vi "SuperScale - 2-17-2012 (SubVI).vi"(0 "Measured Signals":dbl[](array[numeric]), 11 "Error Input":errorcluster, 13 "Scale Reference":refnum<vi>) -> (4 "Scaled Values":dbl[](array[numeric]), 15 "Scale Error":errorcluster)   [LabVIEW 2011]
uses:
  nilvaiu.dll
  C:/Program Files (x86)/National Instruments/LabVIEW 2011/resource/objmgr/daqmx.rc
panel:
  in  "Scale Template":T1={"Channel Select"=0, "Clear/Reset Scales"=FALSE, "Channel #"=["0", "1", "2"], "Scale Names"=["a", "b", "c"], "Set?"=[FALSE, FALSE, FALSE, FALSE, FALSE, FALSE], "HI/LO Setpoints"=[1.0, 0.0, 1.0, 0.0, 1.0, 0.0], "Units"=["vdc", "vdc", "vdc"], "HI/LO Signals"=[1.0, 0.0, 1.0, 0.0, 1.0, 0.0], "Slope/Intercept"=[1.0, 0.0, 1.0, 0.0, 1.0, 0.0], "IN/OUT Values"=[1.0, 1.0, 2.0, 2.0, 3.0, 3.0], "Sim Signals?"=FALSE, "Sim. Signal"=0.0} {"Sim. Signal" format="%#.3p"; "Channel Select" min=0 step=1; "Slope/Intercept" format="%#.3p"; "HI/LO Setpoints" format="%#.3p"; "IN/OUT Values" format="%#.3p"; "HI/LO Signals" format="%#.3p"}
  # "Super Scale SubVI\nCreated by Blake Otting - Ecolab - 2011"
  # "Instructions:\n1) Create the scale interface below by right-clicking on the Scale Template Input of this SubVI (from your main program) and creating a control.\n2) Create a Reference by right-clicking the on scale interface cluster created in step one.\n3) Connect this Reference to the input of this SubVI along with the Measured (Raw) Signals Array."
  # "Scale Template"
  # "OUTPUTS"
  # "INPUTS"
  # "Ch.\n#"
  # "Scale\nName"
  # "Set\nValues?"
  # "Channel\nSelect"
  # "Scaled"
  # "Pre-Scaled"
  # "Scaling Result"
  # "Values"
  # "Units"
  # "Values"
  # "HI"
  # "Slope"
  # "IN"
  # "LO"
  # "Intercept"
  # "OUT"
  # "HI"
  # "Slope"
  # "IN"
  # "LO"
  # "Intercept"
  # "OUT"
  # "HI"
  # "Slope"
  # "IN"
  # "LO"
  # "Intercept"
  # "OUT"
  # "HI"
  # "Slope"
  # "IN"
  # "LO"
  # "Intercept"
  # "OUT"
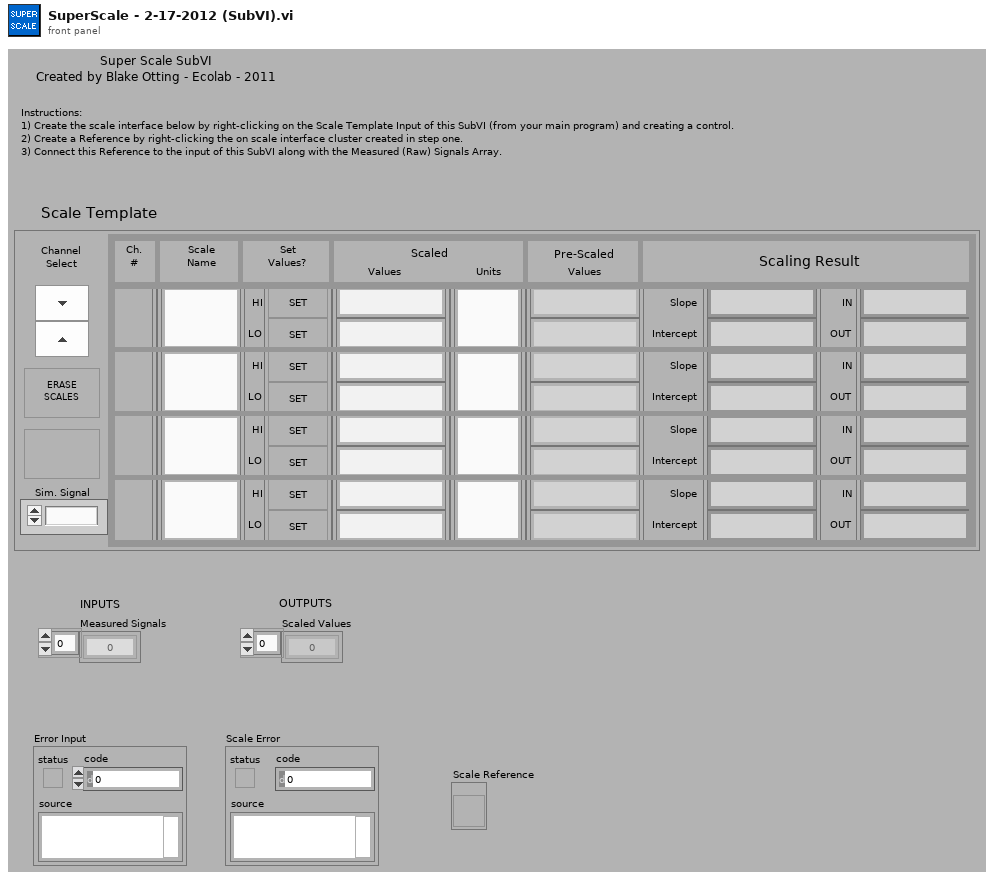
[diagram p1: front panel]
types:
  T1 = cluster{"Channel Select":i32, "Clear/Reset Scales":bool, "Channel #":string[], "Scale Names":string[], "Set?":bool[], "HI/LO Setpoints":dbl[], "Units":string[], "HI/LO Signals":dbl[], "Slope/Intercept":dbl[], "IN/OUT Values":dbl[], "Sim Signals?":bool, "Sim. Signal":dbl}
  T2 = enum16{"open", "replace", "create", "open or create", "replace or create", "replace or create with confirmation"}
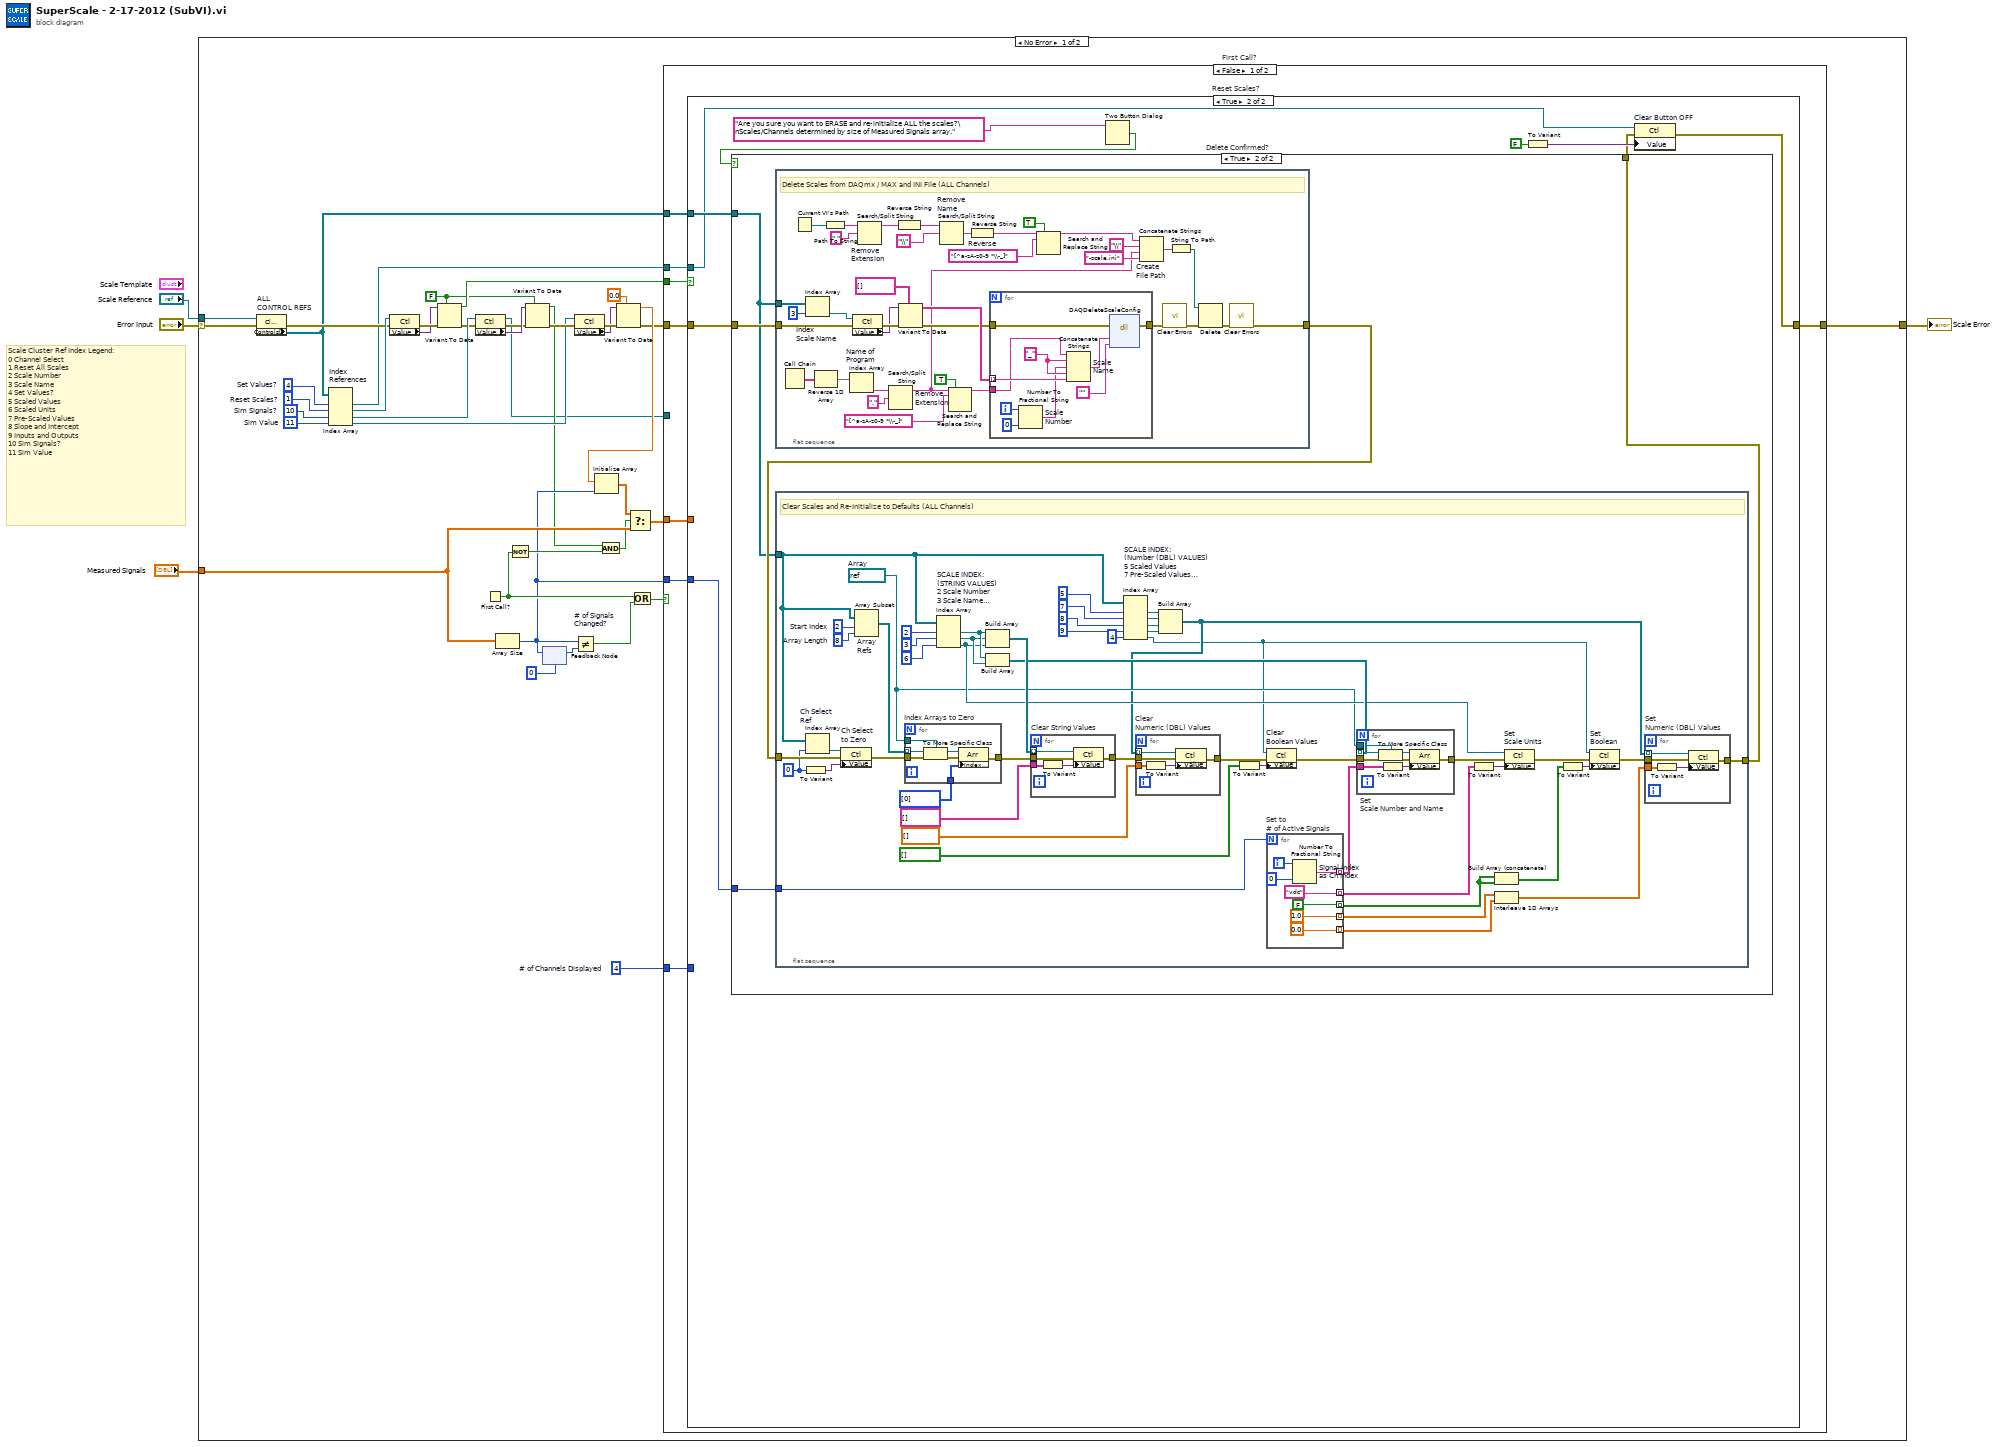
[diagram p0: block diagram]
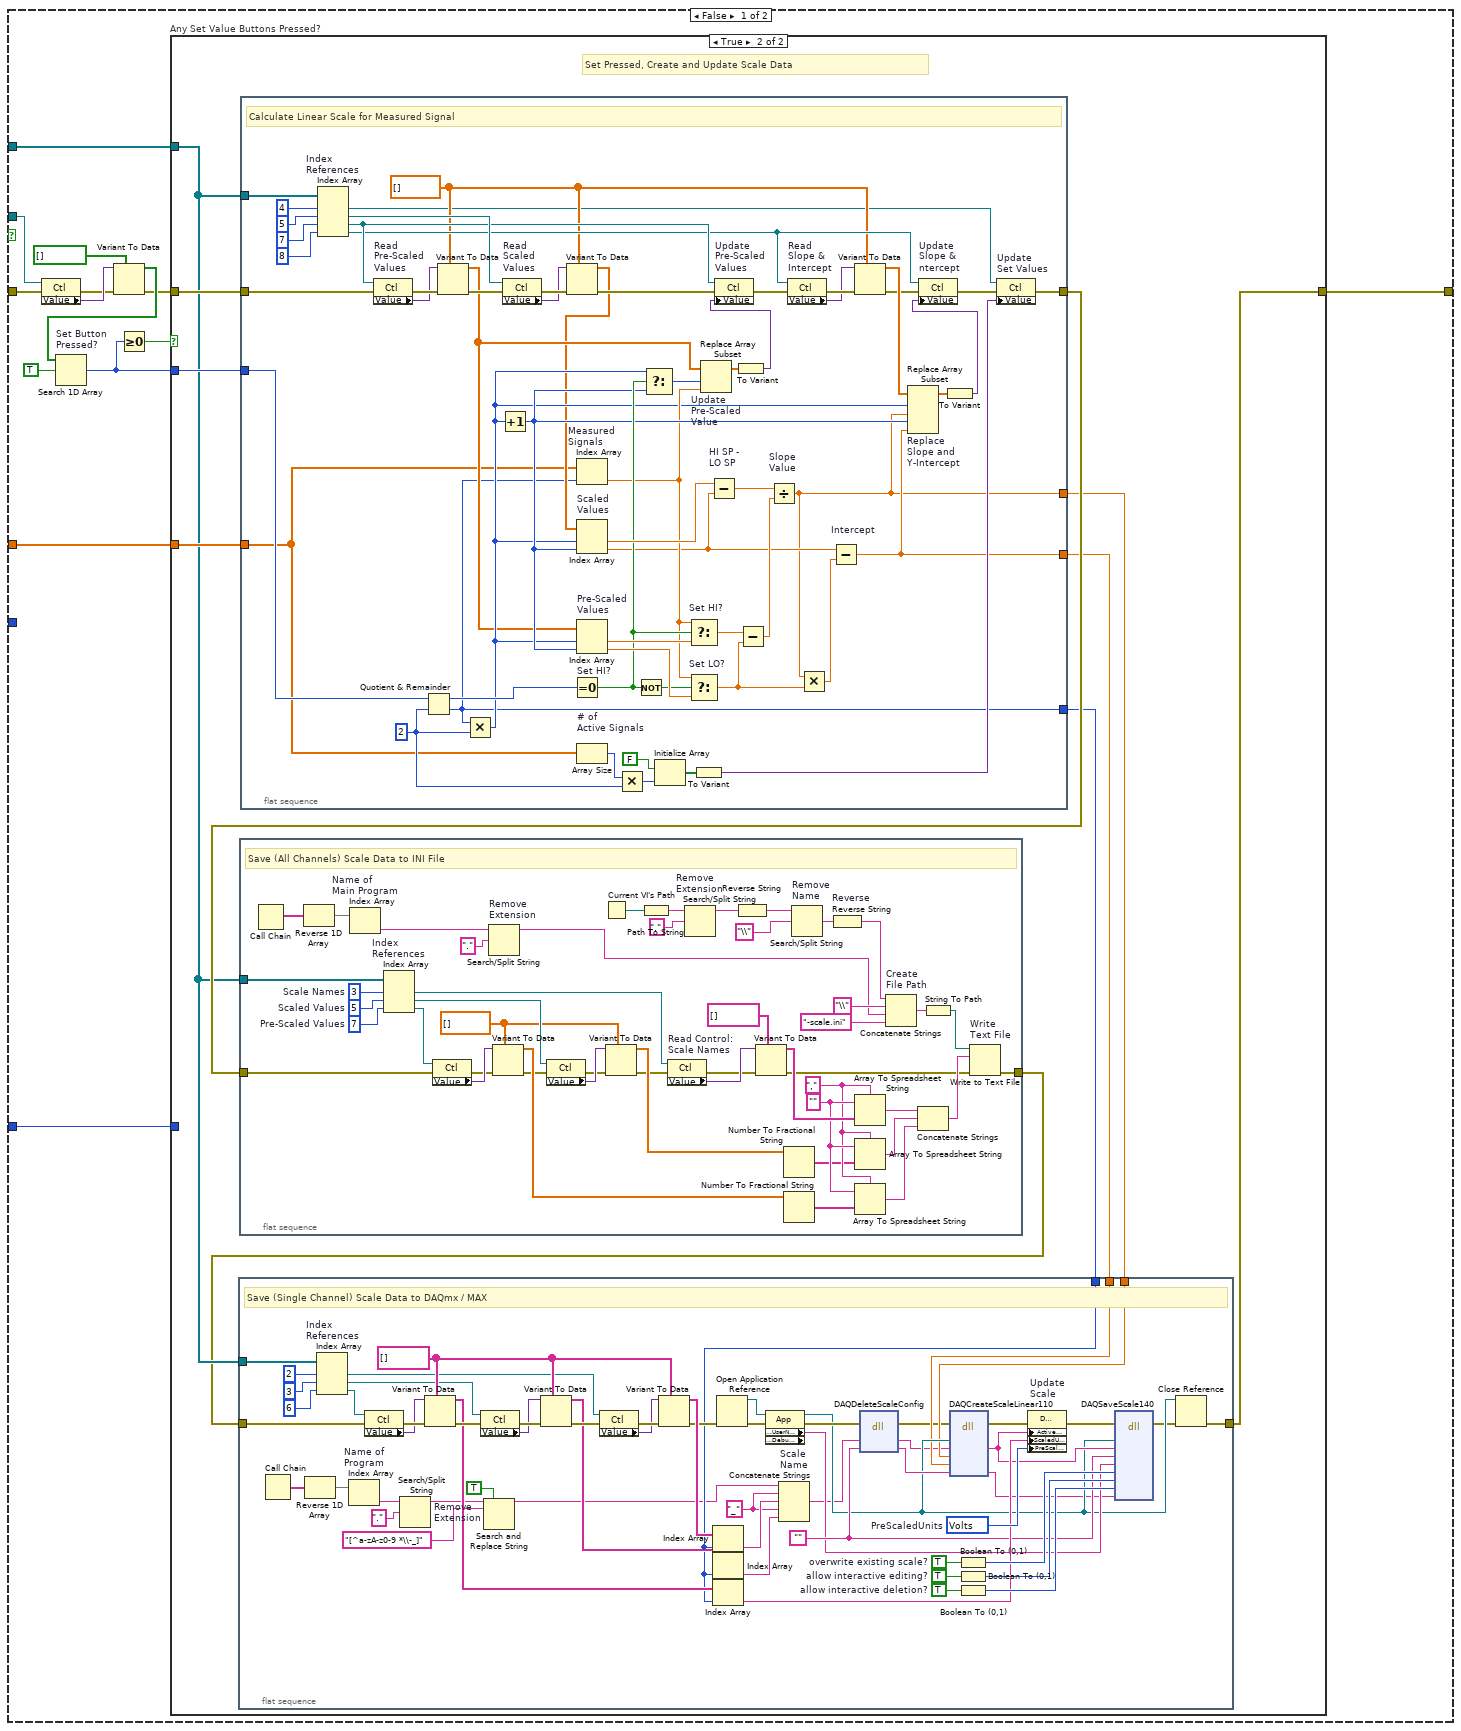
[diagram p2: hidden frame]
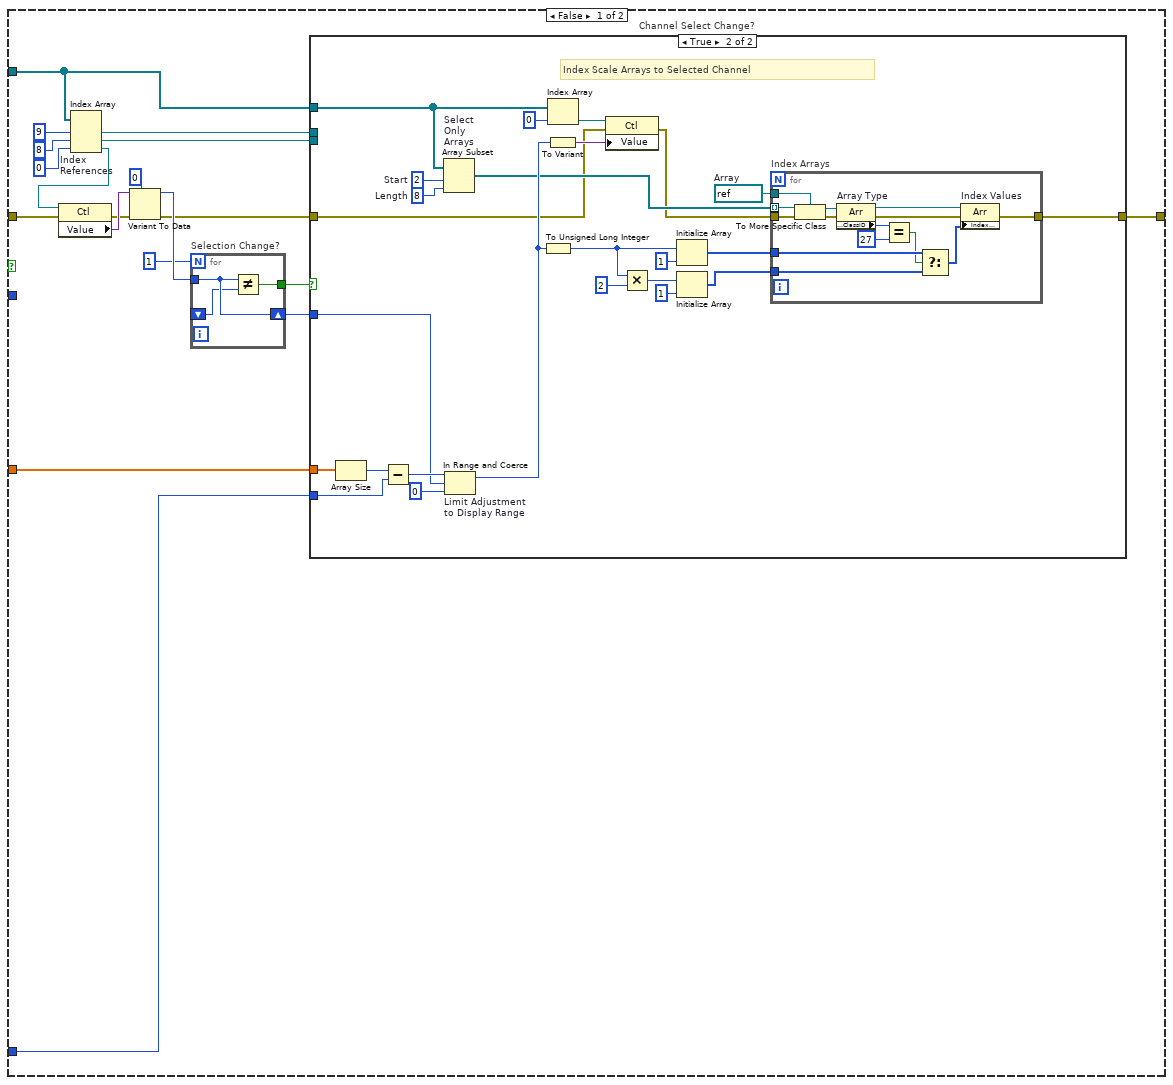
[diagram p3: hidden frame]
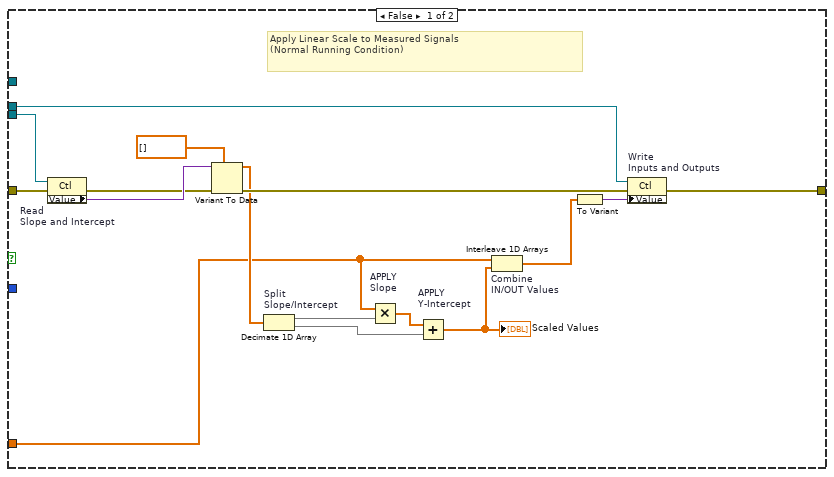
[diagram p4: hidden frame]
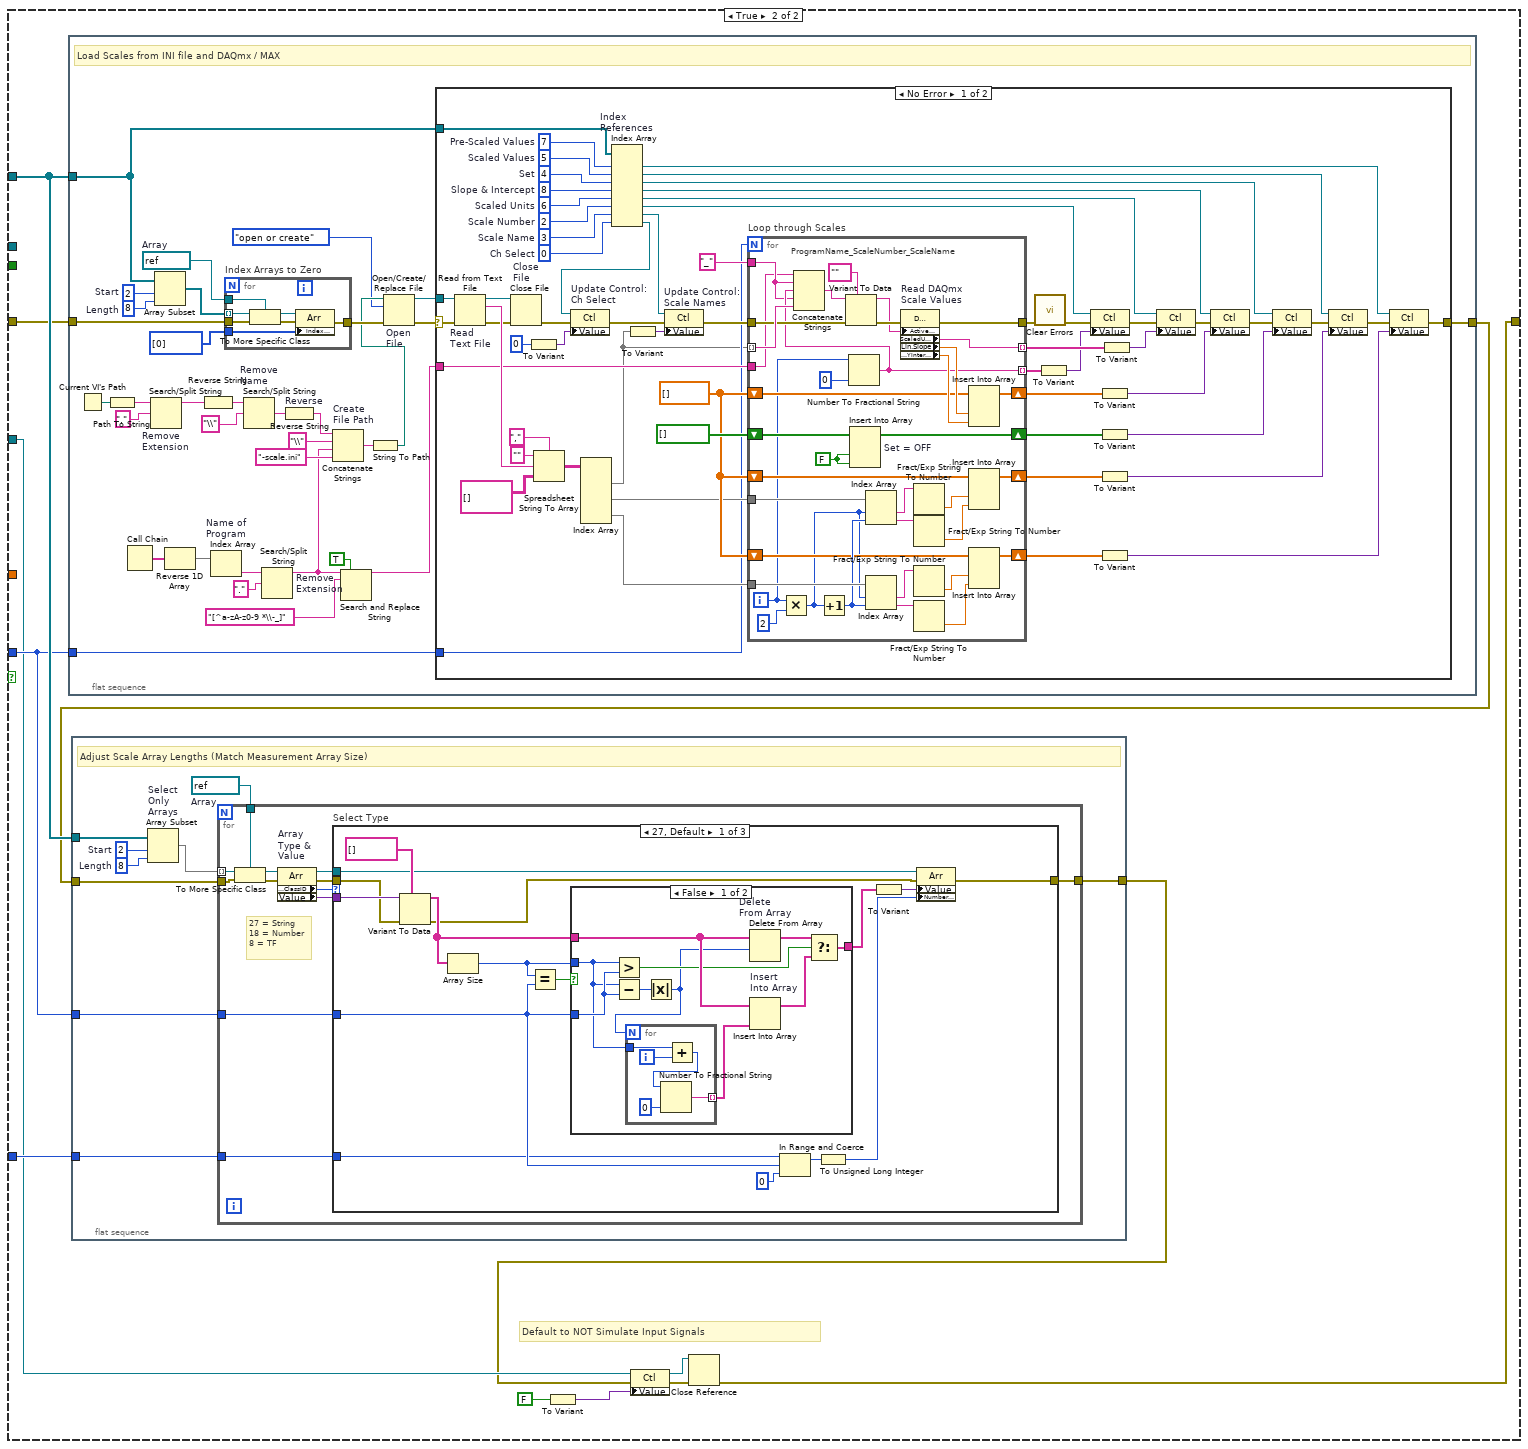
[diagram p6: hidden frame]
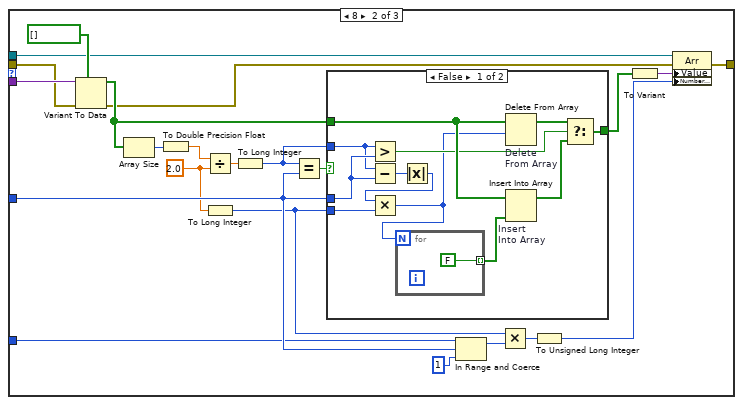
[diagram p8: hidden frame]
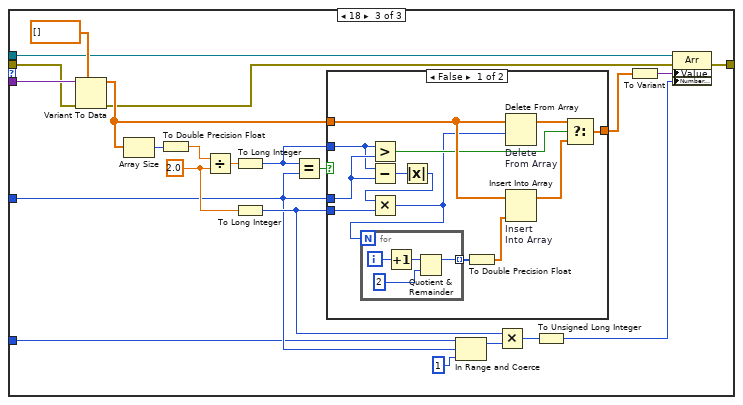
[diagram p10: hidden frame]
diagram:
  # "Scale Cluster Ref Index Legend:\n0 Channel Select\n1 Reset All Scales\n2 Scale Number\n3 Scale Name\n4 Set Values?\n5 Scaled Values\n6 Scaled Units\n7 Pre-Scaled Values\n8 Slope and Intercept\n9 Inputs and Outputs\n10 Sim Signals?\n11 Sim Value"
  n1 = case shown="No Error" "Error Input" {
    selector: "Error Input" -> [w28 w748]
    tunnel: "Scale Reference" -> [w38 _]
    tunnel: "Measured Signals" -> [w25 _]
    tunnel: [w29 w748] -> w3
    frame No Error {
      w19 = 11  # Sim Value
      w20 = 10  # Sim Signals?
      w30 = 4  # Set Values?
      w36 = 4  # # of Channels Displayed
      w14 = FALSE
      w44 = 1  # Reset Scales?
      n2 = property on="ALL\nCONTROL REFS" class="Clust (strict)"(reference=w38, error in=w28) -> (error out=w40:errorcluster, "Controls[]"=w37:refnum<vi>[])  [unwired: 1 out]
      n3 = Index Array "Index\nReferences"(array=w37, index #1=w30, index #2=w44, index #3=w20, index #4=w19) -> (element #1=w31:refnum<vi>, element #2=w43:refnum<vi>, element #3=w18:refnum<vi>, element #4=w8:refnum<vi>)
      n4 = property class="Ctl"(reference=w43, error in=w40) -> (error out=w42:errorcluster, "Value"=w41:variant)  [unwired: 1 out]
      n5 = Variant To Data(error in=w42, type=w14, Variant=w41) -> (data=w39:bool, error out=w17:errorcluster)
      n6 = property class="Ctl"(reference=w18, error in=w17) -> (reference out=w5:refnum<vi>, error out=w15:errorcluster, "Value"=w16:variant)
      n7 = First Call?() -> (First Call?: T/F=w26:bool)
      n8 = Array Size(array=w25) -> (size(s)=w23:i32)
      n9 = Not(x=w26) -> (.not. x?=w27:bool)
      n10 = Variant To Data(error in=w15, type=w14, Variant=w16) -> (data=w6:bool, error out=w9:errorcluster)
      n11 = feedback #1(0) -> (w34:i32)
      n12 = feedback-in #1(w23) -> ()
      n13 = Not Equal? "# of Signals\nChanged?"(x=w23, y=w34) -> (x != y?=w33:bool)
      n14 = property class="Ctl"(reference=w8, error in=w9) -> (error out=w13:errorcluster, "Value"=w7:variant)  [unwired: 1 out]
      n15 = And(x=w6, y=w27) -> (x .and. y?=w21:bool)
      n16 = Variant To Data(error in=w13, type=0.0 ("Simulated Signal"), Variant=w7) -> (data=w11:dbl, error out=w10:errorcluster)
      n17 = Initialize Array(w11, w23) -> (w22:dbl[])
      n18 = Select(t=w22, s=w21, f=w25) -> (s? t:f=w24:dbl[])
      n19 = Or(x=w26, y=w33) -> (x .or. y?=w32:bool)
      n20 = case "First Call?" shown="False" w32 {
        tunnel: w24 -> [w52 _]
        tunnel: w39 -> [w51 _]
        tunnel: w37 -> [w47 w480]
        tunnel: w10 -> [w50 w479]
        tunnel: [w49 w470] -> w29
        tunnel: w36 -> [w48 w478]
        tunnel: w23 -> [w46 w476]
        tunnel: w31 -> [w45 _]
        tunnel: w5 -> [_ w475]
        frame False {
          n21 = case "Reset Scales?" shown="True" w51 {
            tunnel: w47 -> [w55 w321]
            tunnel: w52 -> [w60 _]
            tunnel: w50 -> [w57 w320]
            tunnel: [w56 w325] -> w49
            tunnel: w48 -> [w54 _]
            tunnel: w46 -> [_ w319]
            tunnel: w45 -> [w53 w318]
            frame False {
              n22 = property class="Ctl"(reference=w53, error in=w57) -> (error out=w59:errorcluster, "Value"=w65:variant)  [unwired: 1 out]
              n23 = Variant To Data(error in=w59, type=bool[] [], Variant=w65) -> (data=w63:bool[], error out=w58:errorcluster)
              n24 = Search 1D Array "Set Button\nPressed?"(1D array=w63, element=TRUE) -> (index of element=w61:i32)  [unwired: 1 in]
              n25 = Greater Or Equal To 0?(x=w61) -> (x >= 0?=w62:bool)
              n26 = case "Any Set Value Buttons Pressed?" shown="True" w62 {
                tunnel: w55 -> [w73 w145]
                tunnel: w61 -> [_ w153]
                tunnel: w60 -> [w78 w152]
                tunnel: w58 -> [w77 w151]
                tunnel: [w76 w149] -> w56
                tunnel: w54 -> [w72 _]
                frame False {
                  n27 = Index Array "Index\nReferences"(array=w73, index #1=9, index #2=8, index #3=0) -> (element #1=w68:refnum<vi>, element #2=w71:refnum<vi>, element #3=w74:refnum<vi>)
                  n28 = property class="Ctl"(reference=w74, error in=w77) -> (error out=w83:errorcluster, "Value"=w85:variant)  [unwired: 1 out]
                  n29 = Variant To Data(error in=w83, type=0, Variant=w85) -> (data=w82:i32, error out=w67:errorcluster)
                  n30 = for "Selection Change?" {
                    N: 1 -> [_]
                    tunnel: w82 -> [w143]
                    shift-right: [w143] -> w80
                    shift-left: _ -> [w142]
                    tunnel: [w141] -> w79
                    n31 = Not Equal?(x=w143, y=w142) -> (x != y?=w141:bool)
                  }
                  n32 = case "Channel Select Change?" shown="True" w79 {
                    tunnel: w80 -> [_ w123]
                    tunnel: w67 -> [w101 w103]
                    tunnel: w73 -> [_ w109]
                    tunnel: w78 -> [w88 w122]
                    tunnel: [w100 w104] -> w76
                    tunnel: w72 -> [_ w120]
                    tunnel: w71 -> [w87 _]
                    tunnel: w68 -> [w86 _]
                    frame False {
                      # "Apply Linear Scale to Measured Signals\n(Normal Running Condition)"
                      n33 = property on="Read\nSlope and Intercept" class="Ctl"(reference=w87, error in=w101) -> (error out=w98:errorcluster, "Value"=w99:variant)  [unwired: 1 out]
                      n34 = Variant To Data(error in=w98, type=dbl[] [], Variant=w99) -> (data=w89:dbl[], error out=w90:errorcluster)
                      n35 = Decimate 1D Array "Split\nSlope/Intercept"(w89) -> (w94:dbl[], w95:dbl[])
                      n36 = Multiply "APPLY\nSlope"(x=w88, y=w94) -> (x*y=w96:dbl[])
                      n37 = Add "APPLY\nY-Intercept"(x=w96, y=w95) -> (x+y=w93:dbl[])
                      "Scaled Values" <- w93
                      n38 = Interleave 1D Arrays "Combine\nIN/OUT Values"(w88, w93) -> (w91:dbl[])
                      n39 = To Variant(anything=w91) -> (Variant=w92:variant)
                      n40 = property on="Write\nInputs and Outputs" class="Ctl"(reference=w86, error in=w90, "Value"=w92) -> (error out=w100:errorcluster)  [unwired: 1 out]
                    }
                    frame True {
                      w111 = 8  # Length
                      w110 = 2  # Start
                      w108 = refnum<vi> refnum  # Array
                      # "Index Scale Arrays to Selected Channel"
                      n41 = Array Size(array=w122) -> (size(s)=w121:i32)
                      n42 = Subtract(x=w121, y=w120) -> (x-y=w124:i32)
                      n43 = Array Subset "Select\nOnly \nArrays"(array=w109, index=w110, length=w111) -> (w107:refnum<vi>[])
                      n44 = In Range and Coerce "Limit Adjustment\nto Display Range"(upper limit=w124, x=w123, lower limit=0) -> (coerced(x)=w117:i32)  [unwired: 1 out]
                      n45 = To Unsigned Long Integer(number=w117) -> (unsigned 32bit integer=w114:u32)
                      n46 = Index Array(array=w109, index=0) -> (element=w118:refnum<vi>)
                      n47 = To Variant(anything=w117) -> (Variant=w116:variant)
                      n48 = property class="Ctl"(reference=w118, error in=w103, "Value"=w116) -> (error out=w102:errorcluster)  [unwired: 1 out]
                      n49 = Multiply(x=w114, y=u32 2) -> (x*y=w112:u32)
                      n50 = Initialize Array(w114, 1 ("dimension size")) -> (w106:u32[])
                      n51 = Initialize Array(w112, 1 ("dimension size")) -> (w105:u32[])
                      n52 = for "Index Arrays" {
                        tunnel: w107 -> [w140] mode=indexing
                        tunnel: [w127] -> w104
                        tunnel: w108 -> [w139]
                        tunnel: w102 -> [w138]
                        tunnel: w106 -> [w137]
                        tunnel: w105 -> [w136]
                        n53 = To More Specific Class(target class=w139, reference=w140, error in=w138) -> (specific class reference=w132:refnum<vi>, error out=w133:errorcluster)
                        n54 = property on="Array Type" class="Arr"(reference=w132, error in=w133) -> (reference out=w131:refnum<vi>, error out=w130:errorcluster, "Array Element.ClassID"=w134:u32)
                        n55 = Equal?(x=w134, y=u32 27) -> (x = y?=w128:bool)
                        n56 = Select(t=w137, s=w128, f=w136) -> (s? t:f=w129:u32[])
                        n57 = property on="Index Values" class="Arr"(reference=w131, error in=w130, "Index Values"=w129) -> (error out=w127:errorcluster)  [unwired: 1 out]
                      }
                    }
                  }
                }
                frame True {
                  # "Set Pressed, Create and Update Scale Data"
                  n58 = flat-sequence {
                    tunnel: w145 -> [w240]
                    tunnel: w147 -> [w223]
                    tunnel: w148 -> [w222]
                    tunnel: [w229] -> w149
                    tunnel: w144 -> [w228]
                    tunnel: w146 -> [w221]
                    frame #0 {
                      w254 = string[] []
                      w268 = TRUE  # allow interactive deletion?
                      w267 = TRUE  # allow interactive editing?
                      w266 = TRUE  # overwrite existing scale?
                      w269 = 10348 items=["Volts"=10348, "Amps"=10342, "Deg F"=10144, "Deg C"=10143, "Deg R"=10145, "Kelvins"=10325, "Strain"=10299, "Ohms"=10384, "Hz"=10373, "Seconds"=10364, "Meters"=10219, "Inches"=10379, "Degrees"=10146, "Radians"=10273, "g"=10186, "m/s^2"=12470, "Pascals"=10081, "Newtons"=15875, "Pounds"=15876, "kgf"=15877, "psi"=15879, "bar"=15880, "Nm"=15881, "oz-in"=15882, "lb-in"=15883, "lb-ft"=15884, "Volts/Volt"=15896, "mVolts/Volt"=15897, "From TEDS"=12516]  # PreScaledUnits
                      w238 = ""
                      w234 = "_"
                      # "Save (Single Channel) Scale Data to DAQmx / MAX"
                      n59 = Call Chain() -> (call chain=w225:string[])
                      n60 = Reverse 1D Array(array=w225) -> (reversed array=w224:string[])
                      n61 = Index Array "Index\nReferences"(array=w240, index #1=2, index #2=3, index #3=6) -> (element #1=w251:refnum<vi>, element #2=w250:refnum<vi>, element #3=w249:refnum<vi>)
                      n62 = Index Array "Name of\nProgram"(array=w224) -> (element=w226:string)  [unwired: 1 in]
                      n63 = property class="Ctl"(reference=w249, error in=w228) -> (error out=w259:errorcluster, "Value"=w232:variant)  [unwired: 1 out]
                      n64 = Search/Split String "Remove \nExtension"(string=w226, search string/char (-)=".") -> (substring before match=w213:string)  [unwired: 1 in, 2 out]
                      n65 = Variant To Data(error in=w259, type=w254, Variant=w232) -> (data=w246:string[], error out=w258:errorcluster)
                      n66 = property class="Ctl"(reference=w250, error in=w258) -> (error out=w257:errorcluster, "Value"=w253:variant)  [unwired: 1 out]
                      n67 = Search and Replace String(replace all?=TRUE ("replace all? (F)"), input string=w213, search string="[^a-zA-z0-9 *\\-_]") -> (result string=w214:string)  [unwired: 5 in, 3 out]
                      n68 = Variant To Data(error in=w257, type=w254, Variant=w253) -> (data=w247:string[], error out=w256:errorcluster)
                      n69 = property class="Ctl"(reference=w251, error in=w256) -> (error out=w255:errorcluster, "Value"=w252:variant)  [unwired: 1 out]
                      n70 = Variant To Data(error in=w255, type=w254, Variant=w252) -> (data=w248:string[], error out=w236:errorcluster)
                      n71 = Index Array(array=w248, index=w221) -> (element=w245:string)
                      n72 = Index Array(array=w247, index=w221) -> (element=w244:string)
                      n73 = Index Array(array=w246, index=w221) -> (element=w243:string)
                      n74 = Open Application Reference(8:w236) -> (0:w235:errorcluster, 3:w242:refnum<vi>)  [unwired: 3 in]
                      n75 = property class="App" props=["App.UserName", "App.DebugName"](reference=w242, error in=w235) -> (reference out=w231:refnum<vi>, error out=w237:errorcluster, "App.UserName"=w233:string)  [unwired: 1 out]
                      n76 = Concatenate Strings "Scale\nName"(w214, w234, w245, w234, w244) -> (w216:string)
                      n77 = dll-call lib="nilvaiu.dll" fn="DAQDeleteScaleConfig" label="Delete\nScale"(error in=w237, "scaleName"=w216, "extendedErrorInfo"=w238) -> (error out=w220:errorcluster, "scaleName"=w217:string, "extendedErrorInfo"=w239:string)  [unwired: 3 in, 1 out]
                      n78 = dll-call lib="nilvaiu.*" fn="DAQCreateScaleLinear110" label="Create\nScale"(error in=w220, "This Application"=w231, "name"=w217, "slope"=w222, "yIntercept"=w223, "exterr"=w239) -> (error out=w211:errorcluster, "name"=w241:string, "exterr"=w218:string)  [unwired: 6 in, 1 out]
                      n79 = Boolean To (0,1)(Boolean=w266) -> (0, 1=w265:i16)
                      n80 = Boolean To (0,1)(Boolean=w267) -> (0, 1=w264:i16)
                      n81 = Boolean To (0,1)(Boolean=w268) -> (0, 1=w263:i16)
                      n82 = property on="Update\nScale" class="DAQmx Scale"(error in=w211, "Active Scale"=w241, "ScaledUnits"=w243, "PreScaledUnits"=w269) -> (error out=w219:errorcluster)  [unwired: 1 in, 1 out]
                      n83 = dll-call lib="nilvaiu.*" fn="DAQSaveScale140" label="Save\nScale"(error in=w219, "This Application"=w231, "scaleName"=w241, "saveAs"=w238, "author"=w233, "overwriteMode"=w265, "allowInteractiveEditing?"=w264, "allowInteractiveDeletion?"=w263, "extendedErrorInfo"=w218) -> (error out=w230:errorcluster)  [unwired: 11 in, 1 out]
                      n84 = Close Reference(reference=w231, error in (no error)=w230) -> (error out=w229:errorcluster)
                    }
                  }
                  n85 = flat-sequence {
                    tunnel: w145 -> [w317]
                    tunnel: w150 -> [w316]
                    tunnel: [w315] -> w144
                    frame #0 {
                      w289 = 5  # Scaled Values
                      w290 = 3  # Scale Names
                      w288 = 7  # Pre-Scaled Values
                      w277 = dbl[] [] ("array 2")
                      w302 = "" ("format string")
                      w300 = ","
                      # "Save (All Channels) Scale Data to INI File"
                      n86 = Call Chain() -> (call chain=w273:string[])
                      n87 = Reverse 1D Array(array=w273) -> (reversed array=w272:string[])
                      n88 = Index Array "Name of\nMain Program"(array=w272) -> (element=w274:string)  [unwired: 1 in]
                      n89 = Index Array "Index\nReferences"(array=w317, index #1=w290, index #2=w289, index #3=w288) -> (element #1=w293:refnum<vi>, element #2=w292:refnum<vi>, element #3=w291:refnum<vi>)
                      n90 = property on="Read Control:\nPre-Scaled" class="Ctl"(reference=w291, error in=w316) -> (error out=w310:errorcluster, "Value"=w311:variant)  [unwired: 1 out]
                      n91 = Search/Split String "Remove \nExtension"(string=w274, search string/char (-)=".") -> (substring before match=w271:string)  [unwired: 1 in, 2 out]
                      n92 = Variant To Data(error in=w310, type=w277, Variant=w311) -> (data=w313:dbl[], error out=w312:errorcluster)
                      n93 = property on="Read Control:\nScaled" class="Ctl"(reference=w292, error in=w312) -> (error out=w307:errorcluster, "Value"=w309:variant)  [unwired: 1 out]
                      n94 = Current VI's Path() -> (path=w286:path)
                      n95 = Variant To Data(error in=w307, type=w277, Variant=w309) -> (data=w314:dbl[], error out=w308:errorcluster)
                      n96 = Path To String(path=w286) -> (string=w281:string)
                      n97 = property on="Read Control:\nScale Names" class="Ctl"(reference=w293, error in=w308) -> (error out=w294:errorcluster, "Value"=w296:variant)  [unwired: 1 out]
                      n98 = Search/Split String "Remove \nExtension"(string=w281, search string/char (-)=".") -> (substring before match=w282:string)  [unwired: 1 in, 2 out]
                      n99 = Reverse String ("Reverse")(1:w282) -> (0:w283:string)
                      n100 = Variant To Data(error in=w294, type=string[] [], Variant=w296) -> (data=w305:string[], error out=w304:errorcluster)
                      n101 = Number To Fractional String(number=w314) -> (F-format string=w299:string[])  [unwired: 3 in]
                      n102 = Number To Fractional String(number=w313) -> (F-format string=w303:string[])  [unwired: 3 in]
                      n103 = Search/Split String "Remove\nName"(string=w283, search string/char (-)="\\") -> (match + rest of string=w285:string)  [unwired: 1 in, 2 out]
                      n104 = Reverse String "Reverse"(1:w285) -> (0:w270:string)
                      n105 = Array To Spreadsheet String(delimiter (Tab)=w300, array=w305, 3:w302) -> (spreadsheet string=w297:string)
                      n106 = Array To Spreadsheet String(delimiter (Tab)=w300, array=w299, 3:w302) -> (spreadsheet string=w298:string)
                      n107 = Array To Spreadsheet String(delimiter (Tab)=w300, array=w303, 3:w302) -> (spreadsheet string=w301:string)
                      n108 = Concatenate Strings "Create\nFile Path"(w270, "\\", w271, "-scale.ini") -> (w279:string)
                      n109 = Concatenate Strings(w297, w298, w301) -> (w306:string)
                      n110 = String To Path(string=w279) -> (path=w278:path)
                      n111 = Write to Text File "Write\nText File"(file (use dialog)=w278, text=w306, error in=w304) -> (error out=w315:errorcluster)  [unwired: 1 in, 2 out]
                    }
                  }
                  n112 = flat-sequence {
                    tunnel: w153 -> [w191]
                    tunnel: w152 -> [w160]
                    tunnel: w151 -> [w159]
                    tunnel: [w173] -> w150
                    tunnel: [w154] -> w148
                    tunnel: [w162] -> w147
                    tunnel: [w161] -> w146
                    tunnel: w145 -> [w157]
                    frame #0 {
                      w163 = dbl[] []
                      w166 = 2
                      # "Calculate Linear Scale for Measured Signal"
                      n113 = Index Array "Index\nReferences"(array=w157, index #1=4, index #2=5, index #3=7, index #4=8) -> (element #1=w158:refnum<vi>, element #2=w183:refnum<vi>, element #3=w182:refnum<vi>, element #4=w176:refnum<vi>)
                      n114 = property on="Read\nPre-Scaled\nValues" class="Ctl"(reference=w182, error in=w159) -> (error out=w187:errorcluster, "Value"=w186:variant)  [unwired: 1 out]
                      n115 = Quotient & Remainder(x=w191, y=w166) -> (x-y*floor(x/y)=w194:i32, floor(x/y)=w161:i32)
                      n116 = Variant To Data(error in=w187, type=w163, Variant=w186) -> (data=w165:dbl[], error out=w170:errorcluster)
                      n117 = Multiply(x=w161, y=w166) -> (x*y=w167:i32)
                      n118 = Increment(x=w167) -> (x+1=w198:i32)
                      n119 = property on="Read\nScaled\nValues" class="Ctl"(reference=w183, error in=w170) -> (error out=w185:errorcluster, "Value"=w184:variant)  [unwired: 1 out]
                      n120 = Variant To Data(error in=w185, type=w163, Variant=w184) -> (data=w164:dbl[], error out=w169:errorcluster)
                      n121 = Equal To 0? "Set HI?"(x=w194) -> (x = 0?=w199:bool)
                      n122 = Index Array "Measured\nSignals"(array=w160, index=w161) -> (element=w196:dbl)
                      n123 = Index Array "Scaled\nValues"(array=w164, index #1=w167, index #2=w198) -> (element #1=w210:dbl, element #2=w155:dbl)
                      n124 = Index Array "Pre-Scaled\nValues"(array=w165, index #1=w167, index #2=w198) -> (element #1=w209:dbl, element #2=w208:dbl)
                      n125 = Array Size "# of\nActive Signals"(array=w160) -> (size(s)=w195:i32)
                      n126 = Multiply(x=w195, y=w166) -> (x*y=w200:i32)
                      n127 = Not(x=w199) -> (.not. x?=w204:bool)
                      n128 = Select(t=w167, s=w199, f=w198) -> (s? t:f=w197:i32)
                      n129 = Initialize Array(FALSE, w200) -> (w193:bool[])
                      n130 = Select "Set HI?"(t=w196, s=w199, f=w209) -> (s? t:f=w203:dbl)
                      n131 = Select "Set LO?"(t=w196, s=w204, f=w208) -> (s? t:f=w202:dbl)
                      n132 = To Variant(anything=w193) -> (Variant=w192:variant)
                      n133 = Replace Array Subset "Update\nPre-Scaled\nValue"(array=w165, new element=w196, index=w197) -> (w180:dbl[])
                      n134 = Subtract "HI SP -\nLO SP"(x=w210, y=w155) -> (x-y=w205:dbl)
                      n135 = To Variant(anything=w180) -> (Variant=w181:variant)
                      n136 = property on="Update\nPre-Scaled\nValues" class="Ctl"(reference=w182, error in=w169, "Value"=w181) -> (error out=w168:errorcluster)  [unwired: 1 out]
                      n137 = Subtract(x=w203, y=w202) -> (x-y=w206:dbl)
                      n138 = Divide "Slope\nValue"(x=w205, y=w206) -> (x/y=w154:dbl)
                      n139 = property on="Read\nSlope &\nIntercept" class="Ctl"(reference=w176, error in=w168) -> (error out=w178:errorcluster, "Value"=w177:variant)  [unwired: 1 out]
                      n140 = Multiply(x=w154, y=w202) -> (x*y=w207:dbl)
                      n141 = Subtract "Intercept"(x=w155, y=w207) -> (x-y=w162:dbl)
                      n142 = Variant To Data(error in=w178, type=w163, Variant=w177) -> (data=w175:dbl[], error out=w172:errorcluster)
                      n143 = Replace Array Subset "Replace\nSlope and\nY-Intercept"(array=w175, new element #1=w154, index #1=w167, new element #2=w162, index #2=w198) -> (w174:dbl[])
                      n144 = To Variant(anything=w174) -> (Variant=w171:variant)
                      n145 = property on="Update\nSlope & \nntercept" class="Ctl"(reference=w176, error in=w172, "Value"=w171) -> (error out=w179:errorcluster)  [unwired: 1 out]
                      n146 = property on="Update\nSet Values" class="Ctl"(reference=w158, error in=w179, "Value"=w192) -> (error out=w173:errorcluster)  [unwired: 1 out]
                    }
                  }
                }
              }
            }
            frame True {
              n147 = Two Button Dialog(message="Are you sure you want to ERASE and re-initialize ALL the scales?\nScales/Channels determined by size of Measured Signals array.") -> (T button?=w322:bool)  [unwired: 2 in]
              n148 = case "Delete Confirmed?" shown="True" w322 {
                tunnel: w320 -> [w328 w332]
                tunnel: w321 -> [_ w330]
                tunnel: [w328 w333] -> w324
                tunnel: w319 -> [_ w329]
                frame False {
                  # "User Clicked Cancel \n- Do not delete any scale data"
                }
                frame True {
                  n149 = flat-sequence {
                    tunnel: w330 -> [w452]
                    tunnel: w332 -> [w449]
                    tunnel: [w435] -> w331
                    frame #0 {
                      # "Delete Scales from DAQmx / MAX and INI File (ALL Channels)"
                      n150 = Call Chain() -> (call chain=w433:string[])
                      n151 = Current VI's Path() -> (path=w447:path)
                      n152 = Index Array "Index\nScale Name"(array=w452, index=3) -> (element=w453:refnum<vi>)
                      n153 = Reverse 1D Array(array=w433) -> (reversed array=w434:string[])
                      n154 = Path To String(path=w447) -> (string=w442:string)
                      n155 = Index Array "Name of\nProgram"(array=w434) -> (element=w432:string)  [unwired: 1 in]
                      n156 = property class="Ctl"(reference=w453, error in=w449) -> (error out=w457:errorcluster, "Value"=w455:variant)  [unwired: 1 out]
                      n157 = Search/Split String "Remove \nExtension"(string=w442, search string/char (-)=".") -> (substring before match=w443:string)  [unwired: 1 in, 2 out]
                      n158 = Search/Split String "Remove \nExtension"(string=w432, search string/char (-)=".") -> (substring before match=w423:string)  [unwired: 1 in, 2 out]
                      n159 = Reverse String ("Reverse")(1:w443) -> (0:w444:string)
                      n160 = Variant To Data(error in=w457, type=string[] [], Variant=w455) -> (data=w454:string[], error out=w451:errorcluster)
                      n161 = Search/Split String "Remove\nName"(string=w444, search string/char (-)="\\") -> (match + rest of string=w446:string)  [unwired: 1 in, 2 out]
                      n162 = Search and Replace String(replace all?=TRUE ("replace all? (F)"), input string=w423, search string="[^a-zA-z0-9 *\\-_]") -> (result string=w424:string)  [unwired: 5 in, 3 out]
                      n163 = Reverse String "Reverse"(1:w446) -> (0:w427:string)
                      n164 = for {
                        tunnel: w454 -> [w465] mode=indexing
                        tunnel: w451 -> [w462]
                        tunnel: [w461] -> w450
                        tunnel: w424 -> [w459]
                        i -> [w467]
                        w466 = "_"
                        n165 = Number To Fractional String "Scale\nNumber"(number=w467, precision (6)=i16 0) -> (F-format string=w464:string)  [unwired: 2 in]
                        n166 = Concatenate Strings "Scale\nName"(w459, w466, w464, w466, w465) -> (w463:string)
                        n167 = dll-call lib="nilvaiu.dll" fn="DAQDeleteScaleConfig" label="Delete\nScale"(error in=w462, "scaleName"=w463, "extendedErrorInfo"="") -> (error out=w461:errorcluster)  [unwired: 5 in, 1 out]
                      }
                      n168 = Search and Replace String(replace all?=TRUE ("replace all? (F)"), input string=w427, search string="[^a-zA-z0-9 *\\-_]") -> (result string=w428:string)  [unwired: 5 in, 3 out]
                      n169 = Concatenate Strings "Create\nFile Path"(w428, "\\", w423, "-scale.ini") -> (w437:string)
                      n170 = call <vilib>:"Clear Errors.vi"("error in (no error)"=w450) -> ("error out"=w438:errorcluster)  [unwired: 6 in]
                      n171 = String To Path(string=w437) -> (path=w439:path)
                      n172 = Delete(path (use dialog)=w439, error in=w438) -> (error out=w436:errorcluster)  [unwired: 3 in, 2 out]
                      n173 = call <vilib>:"Clear Errors.vi"("error in (no error)"=w436) -> ("error out"=w435:errorcluster)  [unwired: 6 in]
                    }
                  }
                  n174 = flat-sequence {
                    tunnel: [w343] -> w333
                    tunnel: w331 -> [w341]
                    tunnel: w330 -> [w339]
                    tunnel: w329 -> [w340]
                    frame #0 {
                      w337 = 0
                      w344 = refnum<vi> refnum  # Array
                      w383 = 8  # Array Length
                      w385 = 2  # Start Index
                      # "Clear Scales and Re-Initialize to Defaults (ALL Channels)"
                      n175 = To Variant(anything=w337) -> (Variant=w382:variant)
                      n176 = Index Array "Ch Select\nRef"(array=w339, index=w337) -> (element=w338:refnum<vi>)
                      n177 = property on="Ch Select\nto Zero" class="Ctl"(reference=w338, error in=w341, "Value"=w382) -> (error out=w351:errorcluster)  [unwired: 1 out]
                      n178 = Array Subset "Array\nRefs"(array=w339, index=w385, length=w383) -> (w384:refnum<vi>[])
                      n179 = for "Index Arrays to Zero" {
                        tunnel: w384 -> [w422] mode=indexing
                        tunnel: [w420] -> w353
                        tunnel: w344 -> [w419]
                        tunnel: u32[] [0] -> [w418]
                        tunnel: w351 -> [w417]
                        n180 = To More Specific Class(target class=w419, reference=w422, error in=w417) -> (specific class reference=w416:refnum<vi>, error out=w421:errorcluster)
                        n181 = property class="Arr"(reference=w416, error in=w421, "Index Values"=w418) -> (error out=w420:errorcluster)  [unwired: 1 out]
                      }
                      n182 = Index Array "SCALE INDEX:\n(STRING VALUES)\n2 Scale Number\n3 Scale Name\n6 Scaled Units"(array=w339, index #1=2, index #2=3, index #3=6) -> (element #1=w350:refnum<vi>, element #2=w349:refnum<vi>, element #3=w347:refnum<vi>)
                      n183 = Build Array(w350, w349, w347) -> (w381:refnum<vi>[])
                      n184 = Build Array(w350, w349) -> (w367:refnum<vi>[])
                      n185 = for "Clear String Values" {
                        tunnel: w381 -> [w412] mode=indexing
                        tunnel: [w414] -> w355
                        tunnel: string[] [] -> [w413]
                        tunnel: w353 -> [w411]
                        n186 = To Variant(anything=w413) -> (Variant=w415:variant)
                        n187 = property class="Ctl"(reference=w412, error in=w411, "Value"=w415) -> (error out=w414:errorcluster)  [unwired: 1 out]
                      }
                      n188 = Index Array "SCALE INDEX:\n(Number (DBL) VALUES)\n5 Scaled Values\n7 Pre-Scaled Values\n8 Slope and Intercept\n9 Inputs and Outputs"(array=w339, index #1=5, index #2=7, index #3=8, index #4=9, index #5=4 ("index")) -> (element #1=w377:refnum<vi>, element #2=w376:refnum<vi>, element #3=w375:refnum<vi>, element #4=w370:refnum<vi>, element #5=w335:refnum<vi>)
                      n189 = Build Array(w377, w376, w375, w370) -> (w342:refnum<vi>[])
                      n190 = for "Clear\nNumeric (DBL) Values" {
                        tunnel: w342 -> [w407] mode=indexing
                        tunnel: w355 -> [w406]
                        tunnel: dbl[] [] -> [w409]
                        tunnel: [w408] -> w348
                        n191 = To Variant(anything=w409) -> (Variant=w410:variant)
                        n192 = property class="Ctl"(reference=w407, error in=w406, "Value"=w410) -> (error out=w408:errorcluster)  [unwired: 1 out]
                      }
                      n193 = To Variant(anything=bool[] []) -> (Variant=w369:variant)
                      n194 = property on="Clear\nBoolean Values" class="Ctl"(reference=w335, error in=w348, "Value"=w369) -> (error out=w356:errorcluster)  [unwired: 1 out]
                      n195 = for "Set to \n# of Active Signals" {
                        N: w340 -> [_]
                        tunnel: [w403] -> w366 mode=indexing
                        tunnel: ["vdc"] -> w364 mode=indexing
                        tunnel: [FALSE] -> w363 mode=indexing
                        tunnel: [1.0 ("Value")] -> w362 mode=indexing
                        tunnel: [0.0 ("Value")] -> w334 mode=indexing
                        i -> [w404]
                        n196 = Number To Fractional String "Signal Index\nas Ch Index"(number=w404, precision (6)=i16 0) -> (F-format string=w403:string)  [unwired: 2 in]
                      }
                      n197 = for "Set\nScale Number and Name" {
                        tunnel: w367 -> [w392] mode=indexing
                        tunnel: w366 -> [w397]
                        tunnel: [w396] -> w346
                        tunnel: w356 -> [w395]
                        tunnel: w344 -> [w394]
                        n198 = To More Specific Class(target class=w394, reference=w392, error in=w395) -> (specific class reference=w391:refnum<vi>, error out=w393:errorcluster)
                        n199 = To Variant(anything=w397) -> (Variant=w398:variant)
                        n200 = property class="Arr"(reference=w391, error in=w393, "Value"=w398) -> (error out=w396:errorcluster)  [unwired: 1 out]
                      }
                      n201 = To Variant(anything=w364) -> (Variant=w365:variant)
                      n202 = Build Array (concatenate)(w363, w363) -> (w359:bool[])
                      n203 = Interleave 1D Arrays(w362, w334) -> (w361:dbl[])
                      n204 = property on="Set\nScale Units" class="Ctl"(reference=w347, error in=w346, "Value"=w365) -> (error out=w345:errorcluster)  [unwired: 1 out]
                      n205 = To Variant(anything=w359) -> (Variant=w360:variant)
                      n206 = property on="Set\nBoolean" class="Ctl"(reference=w335, error in=w345, "Value"=w360) -> (error out=w358:errorcluster)  [unwired: 1 out]
                      n207 = for "Set\nNumeric (DBL) Values" {
                        tunnel: w342 -> [w387] mode=indexing
                        tunnel: w361 -> [w389]
                        tunnel: w358 -> [w388]
                        tunnel: [w386] -> w343
                        n208 = To Variant(anything=w389) -> (Variant=w390:variant)
                        n209 = property class="Ctl"(reference=w387, error in=w388, "Value"=w390) -> (error out=w386:errorcluster)  [unwired: 1 out]
                      }
                    }
                  }
                }
              }
              n210 = To Variant(anything=FALSE) -> (Variant=w326:variant)
              n211 = property on="Clear Button OFF" class="Ctl"(reference=w318, error in=w324, "Value"=w326) -> (error out=w325:errorcluster)  [unwired: 1 out]
            }
          }
        }
        frame True {
          # "Default to NOT Simulate Input Signals"
          n212 = flat-sequence {
            tunnel: w480 -> [w620]
            tunnel: [w635] -> w477
            tunnel: w479 -> [w622]
            tunnel: w476 -> [w610]
            frame #0 {
              w637 = 8  # Length
              w638 = 2  # Start
              w639 = refnum<vi> refnum  # Array
              # "Load Scales from INI file and DAQmx / MAX"
              n213 = Current VI's Path() -> (path=w627:path)
              n214 = Path To String(path=w627) -> (string=w632:string)
              n215 = Call Chain() -> (call chain=w618:string[])
              n216 = Search/Split String "Remove \nExtension"(string=w632, search string/char (-)=".") -> (substring before match=w631:string)  [unwired: 1 in, 2 out]
              n217 = Array Subset(array=w620, index=w638, length=w637) -> (w636:refnum<vi>[])
              n218 = Reverse 1D Array(array=w618) -> (reversed array=w619:string[])
              n219 = Reverse String ("Reverse")(1:w631) -> (0:w630:string)
              n220 = Index Array "Name of\nProgram"(array=w619) -> (element=w617:string)  [unwired: 1 in]
              n221 = for "Index Arrays to Zero" {
                tunnel: w636 -> [w747] mode=indexing
                tunnel: [w745] -> w640
                tunnel: w639 -> [w744]
                tunnel: u32[] [0] -> [w743]
                tunnel: w622 -> [w742]
                n222 = To More Specific Class(target class=w744, reference=w747, error in=w742) -> (specific class reference=w741:refnum<vi>, error out=w746:errorcluster)
                n223 = property class="Arr"(reference=w741, error in=w746, "Index Values"=w743) -> (error out=w745:errorcluster)  [unwired: 1 out]
              }
              n224 = Search/Split String "Remove\nName"(string=w630, search string/char (-)="\\") -> (match + rest of string=w628:string)  [unwired: 1 in, 2 out]
              n225 = Search/Split String "Remove \nExtension"(string=w617, search string/char (-)=".") -> (substring before match=w613:string)  [unwired: 1 in, 2 out]
              n226 = Reverse String "Reverse"(1:w628) -> (0:w611:string)
              n227 = Concatenate Strings "Create\nFile Path"(w611, "\\", w613, "-scale.ini") -> (w634:string)
              n228 = Search and Replace String(replace all?=TRUE ("replace all? (F)"), input string=w613, search string="[^a-zA-z0-9 *\\-_]") -> (result string=w612:string)  [unwired: 5 in, 3 out]
              n229 = String To Path(string=w634) -> (path=w625:path)
              n230 = Open/Create/Replace File "Open\nFile"(file path (use dialog)=w625, error in=w640, operation (0:open)=T2."open or create") -> (refnum out=w642:refnum<file>, error out=w623:errorcluster)  [unwired: 3 in, 1 out]
              n231 = case shown="No Error" w623 {
                selector: w623 -> [w669 w740]
                tunnel: w642 -> [w676 _]
                tunnel: [w670 w740] -> w635
                tunnel: w620 -> [w653 _]
                tunnel: w612 -> [w645 _]
                tunnel: w610 -> [w644 _]
                frame No Error {
                  w655 = 0  # Ch Select
                  w656 = 7  # Pre-Scaled Values
                  w657 = 5  # Scaled Values
                  w658 = 4  # Set
                  w659 = 8  # Slope & Intercept
                  w660 = 6  # Scaled Units
                  w661 = 2  # Scale Number
                  w662 = 3  # Scale Name
                  w691 = dbl[] [] ("array")
                  n232 = Read from Text File "Read\nText File"(file (use dialog)=w676, error in=w669) -> (refnum out=w675:refnum<file>, text=w681:string, error out=w677:errorcluster)  [unwired: 2 in, 1 out]
                  n233 = Close File "Close\nFile"(refnum=w675, error in=w677) -> (error out=w673:errorcluster)  [unwired: 1 out]
                  n234 = To Variant(anything=0) -> (Variant=w671:variant)
                  n235 = Spreadsheet String To Array(delimiter (Tab)=",", format string="", spreadsheet string=w681, array type (2D Dbl)=string[][] [] ("appended array")) -> (array=w680:string[][])
                  n236 = Index Array(array=w680) -> (element #1=w643:string[], element #2=w679:string[], element #3=w678:string[])  [unwired: 6 in]
                  n237 = Index Array "Index\nReferences"(array=w653, index #1=w656, index #2=w657, index #3=w658, index #4=w659, index #5=w660, index #6=w661, index #7=w662, index #8=w655) -> (element #1=w646:refnum<vi>, element #2=w647:refnum<vi>, element #3=w648:refnum<vi>, element #4=w649:refnum<vi>, element #5=w650:refnum<vi>, element #6=w651:refnum<vi>, element #7=w652:refnum<vi>, element #8=w654:refnum<vi>)
                  n238 = property on="Update Control:\nCh Select" class="Ctl"(reference=w654, error in=w673, "Value"=w671) -> (error out=w672:errorcluster)  [unwired: 1 out]
                  n239 = To Variant(anything=w643) -> (Variant=w698:variant)
                  n240 = property on="Update Control:\nScale Names" class="Ctl"(reference=w652, error in=w672, "Value"=w698) -> (error out=w697:errorcluster)  [unwired: 1 out]
                  n241 = for "Loop through Scales" {
                    N: w644 -> [_]
                    tunnel: w643 -> [w734] mode=indexing
                    tunnel: [w733] -> w701 mode=indexing
                    shift-right: [w730] -> w699
                    shift-left: w691 -> [w729]
                    tunnel: w697 -> [w710]
                    shift-right: [w726] -> w694
                    shift-left: bool[] [] -> [w727]
                    shift-right: [w724] -> w689
                    shift-left: w691 -> [w725]
                    tunnel: w679 -> [w723]
                    tunnel: w678 -> [w718]
                    shift-right: [w711] -> w688
                    shift-left: w691 -> [w712]
                    tunnel: [w709] -> w667 mode=indexing
                    tunnel: [w708] -> w665
                    tunnel: "_" -> [w707]
                    tunnel: w645 -> [w706]
                    i -> [w705]
                    w728 = FALSE
                    # "ProgramName_ScaleNumber_ScaleName"
                    n242 = Multiply(x=w705, y=2) -> (x*y=w703:i32)
                    n243 = Increment(x=w703) -> (x+1=w717:i32)
                    n244 = Number To Fractional String(number=w705, precision (6)=i16 0) -> (F-format string=w709:string)  [unwired: 2 in]
                    n245 = Concatenate Strings(w706, w707, w709, w707, w734) -> (w737:string)
                    n246 = Variant To Data(error in=w710, type=tag "" ("ActiveScale"), Variant=w737) -> (data=w735:tag, error out=w736:errorcluster)
                    n247 = Insert Into Array "Set = OFF"(array=w727, new element #1=w728, new element #2=w728) -> (w726:bool[])  [unwired: 1 in]
                    n248 = Index Array(array=w723, index #1=w703, index #2=w717) -> (element #1=w722:string, element #2=w719:string)
                    n249 = Index Array(array=w718, index #1=w703, index #2=w717) -> (element #1=w716:string, element #2=w715:string)
                    n250 = property on="Read DAQmx\nScale Values" class="DAQmx Scale"(error in=w736, "Active Scale"=w735) -> (error out=w708:errorcluster, "ScaledUnits"=w733:string, "Lin.Slope"=w732:dbl, "Lin.YIntercept"=w731:dbl)  [unwired: 1 in, 1 out]
                    n251 = Fract/Exp String To Number(string=w722) -> (number=w721:dbl)  [unwired: 3 in, 1 out]
                    n252 = Fract/Exp String To Number(string=w719) -> (number=w720:dbl)  [unwired: 3 in, 1 out]
                    n253 = Fract/Exp String To Number(string=w716) -> (number=w714:dbl)  [unwired: 3 in, 1 out]
                    n254 = Fract/Exp String To Number(string=w715) -> (number=w713:dbl)  [unwired: 3 in, 1 out]
                    n255 = Insert Into Array(array=w729, new element #1=w732, new element #2=w731) -> (w730:dbl[])  [unwired: 1 in]
                    n256 = Insert Into Array(array=w725, new element #1=w721, new element #2=w720) -> (w724:dbl[])  [unwired: 1 in]
                    n257 = Insert Into Array(array=w712, new element #1=w714, new element #2=w713) -> (w711:dbl[])  [unwired: 1 in]
                  }
                  n258 = call <vilib>:"Clear Errors.vi"("error in (no error)"=w665) -> ("error out"=w664:errorcluster)  [unwired: 6 in]
                  n259 = To Variant(anything=w667) -> (Variant=w668:variant)
                  n260 = property on="Update Control:\nScale Numbers" class="Ctl"(reference=w651, error in=w664, "Value"=w668) -> (error out=w666:errorcluster)  [unwired: 1 out]
                  n261 = To Variant(anything=w699) -> (Variant=w702:variant)
                  n262 = To Variant(anything=w694) -> (Variant=w696:variant)
                  n263 = To Variant(anything=w689) -> (Variant=w687:variant)
                  n264 = To Variant(anything=w688) -> (Variant=w685:variant)
                  n265 = To Variant(anything=w701) -> (Variant=w700:variant)
                  n266 = property on="Update Control:\nScaled Units" class="Ctl"(reference=w650, error in=w666, "Value"=w700) -> (error out=w693:errorcluster)  [unwired: 1 out]
                  n267 = property on="Update Control:\nSlope and Intercept" class="Ctl"(reference=w649, error in=w693, "Value"=w702) -> (error out=w692:errorcluster)  [unwired: 1 out]
                  n268 = property on="Update Control:\nSet Buttons" class="Ctl"(reference=w648, error in=w692, "Value"=w696) -> (error out=w690:errorcluster)  [unwired: 1 out]
                  n269 = property on="Update Control:\nScaled Values" class="Ctl"(reference=w647, error in=w690, "Value"=w687) -> (error out=w686:errorcluster)  [unwired: 1 out]
                  n270 = property on="Update Control:\nPre-Scaled Values" class="Ctl"(reference=w646, error in=w686, "Value"=w685) -> (error out=w670:errorcluster)  [unwired: 1 out]
                }
                frame Error {
                }
              }
            }
          }
          n271 = flat-sequence {
            tunnel: w480 -> [w487]
            tunnel: w476 -> [w486]
            tunnel: w478 -> [w483]
            tunnel: w477 -> [w482]
            tunnel: [w481] -> w473
            frame #0 {
              w484 = refnum<vi> refnum  # Array
              w488 = 8  # Length
              w489 = 2  # Start
              # "Adjust Scale Array Lengths (Match Measurement Array Size)"
              n272 = Array Subset "Select\nOnly \nArrays"(array=w487, index=w489, length=w488) -> (w485:refnum<vi>[])
              n273 = for {
                tunnel: w485 -> [w500] mode=indexing
                tunnel: w484 -> [w499]
                tunnel: w486 -> [w495]
                tunnel: [w493] -> w481
                tunnel: w483 -> [w491]
                tunnel: w482 -> [w490]
                # "27 = String\n18 = Number\n8 = TF"
                n274 = To More Specific Class(target class=w499, reference=w500, error in=w490) -> (specific class reference=w501:refnum<vi>, error out=w492:errorcluster)
                n275 = property on="Array\nType &\nValue" class="Arr"(reference=w501, error in=w492) -> (reference out=w496:refnum<vi>, error out=w494:errorcluster, "Array Element.ClassID"=w497:u32, "Value"=w498:variant)
                n276 = case "Select Type" shown="27, Default" w497 {
                  tunnel: w498 -> [w517 w555 w591]
                  tunnel: w496 -> [w510 w549 w585]
                  tunnel: w495 -> [w508 w543 w573]
                  tunnel: w494 -> [w503 w535 w571]
                  tunnel: [w509 w548 w584] -> w493
                  tunnel: w491 -> [w507 w536 w572]
                  frame 27, Default {
                    n277 = Variant To Data(error in=w503, type=string[] [] ("appended array"), Variant=w517) -> (data=w512:string[], error out=w502:errorcluster)
                    n278 = Array Size(array=w512) -> (size(s)=w511:i32)
                    n279 = Equal?(x=w511, y=w508) -> (x = y?=w515:bool)
                    n280 = case shown="False" w515 {
                      tunnel: w511 -> [w518 _]
                      tunnel: w512 -> [w525 w533]
                      tunnel: w508 -> [w527 _]
                      tunnel: [w523 w533] -> w513
                      frame False {
                        n281 = Greater?(x=w518, y=w527) -> (0:w521:bool)
                        n282 = Subtract(x=w518, y=w527) -> (x-y=w526:i32)
                        n283 = Absolute Value(x=w526) -> (abs(x)=w519:i32)
                        n284 = for {
                          N: w519 -> [_]
                          tunnel: w518 -> [w532]
                          tunnel: [w530] -> w520 mode=indexing
                          i -> [w528]
                          n285 = Add(x=w532, y=w528) -> (x+y=w529:i32)
                          n286 = Number To Fractional String(number=w529, precision (6)=i16 0) -> (F-format string=w530:string)  [unwired: 2 in]
                        }
                        n287 = Delete From Array "Delete \nFrom Array"(array=w525, length=w519) -> (array with subset deleted=w524:string[])  [unwired: 1 in, 1 out]
                        n288 = Insert Into Array "Insert \nInto Array"(array=w525, new element=w520) -> (w522:string[])  [unwired: 1 in]
                        n289 = Select(t=w524, s=w521, f=w522) -> (s? t:f=w523:string[])
                      }
                      frame True {
                      }
                    }
                    n290 = In Range and Coerce(upper limit=w507, x=w508, lower limit=0) -> (coerced(x)=w505:i32)  [unwired: 1 out]
                    n291 = To Unsigned Long Integer(number=w505) -> (unsigned 32bit integer=w504:u32)
                    n292 = To Variant(anything=w513) -> (Variant=w514:variant)
                    n293 = property class="Arr"(reference=w510, error in=w502, "Value"=w514, "Number of Rows"=w504) -> (error out=w509:errorcluster)  [unwired: 1 out]
                  }
                  frame 8 {
                    w540 = 2.0 ("y")
                    n294 = Variant To Data(error in=w535, type=bool[] [] ("appended array"), Variant=w555) -> (data=w550:bool[], error out=w534:errorcluster)
                    n295 = Array Size(array=w550) -> (size(s)=w545:i32)
                    n296 = To Double Precision Float(number=w545) -> (double precision float=w544:dbl)
                    n297 = Divide(x=w544, y=w540) -> (x/y=w542:dbl)
                    n298 = To Long Integer(number=w540) -> (32bit integer=w538:i32)
                    n299 = To Long Integer(number=w542) -> (32bit integer=w541:i32)
                    n300 = Equal?(x=w541, y=w543) -> (x = y?=w553:bool)
                    n301 = case shown="False" w553 {
                      tunnel: w541 -> [w559 _]
                      tunnel: w550 -> [w565 w569]
                      tunnel: w543 -> [w567 _]
                      tunnel: [w563 w569] -> w551
                      tunnel: w538 -> [w557 _]
                      frame False {
                        n302 = Greater?(x=w559, y=w567) -> (0:w561:bool)
                        n303 = Subtract(x=w559, y=w567) -> (x-y=w566:i32)
                        n304 = Absolute Value(x=w566) -> (abs(x)=w558:i32)
                        n305 = Multiply(x=w558, y=w557) -> (x*y=w556:i32)
                        n306 = for {
                          N: w556 -> [_]
                          tunnel: [FALSE] -> w560 mode=indexing
                        }
                        n307 = Delete From Array "Delete \nFrom Array"(array=w565, length=w556) -> (array with subset deleted=w564:bool[])  [unwired: 1 in, 1 out]
                        n308 = Insert Into Array "Insert \nInto Array"(array=w565, new element=w560) -> (w562:bool[])  [unwired: 1 in]
                        n309 = Select(t=w564, s=w561, f=w562) -> (s? t:f=w563:bool[])
                      }
                      frame True {
                      }
                    }
                    n310 = In Range and Coerce(upper limit=w536, x=w543, lower limit=1) -> (coerced(x)=w539:i32)  [unwired: 1 out]
                    n311 = Multiply(x=w538, y=w539) -> (x*y=w537:i32)
                    n312 = To Unsigned Long Integer(number=w537) -> (unsigned 32bit integer=w546:u32)
                    n313 = To Variant(anything=w551) -> (Variant=w552:variant)
                    n314 = property class="Arr"(reference=w549, error in=w534, "Value"=w552, "Number of Rows"=w546) -> (error out=w548:errorcluster)  [unwired: 1 out]
                  }
                  frame 18 {
                    w578 = 2.0 ("y")
                    n315 = Variant To Data(error in=w571, type=dbl[] [] ("appended array"), Variant=w591) -> (data=w586:dbl[], error out=w570:errorcluster)
                    n316 = Array Size(array=w586) -> (size(s)=w582:i32)
                    n317 = To Double Precision Float(number=w582) -> (double precision float=w581:dbl)
                    n318 = Divide(x=w581, y=w578) -> (x/y=w580:dbl)
                    n319 = To Long Integer(number=w580) -> (32bit integer=w579:i32)
                    n320 = To Long Integer(number=w578) -> (32bit integer=w574:i32)
                    n321 = Equal?(x=w579, y=w573) -> (x = y?=w589:bool)
                    n322 = case shown="False" w589 {
                      tunnel: w579 -> [w597 _]
                      tunnel: w586 -> [w602 w609]
                      tunnel: w573 -> [w604 _]
                      tunnel: [w600 w609] -> w587
                      tunnel: w574 -> [w595 _]
                      frame False {
                        n323 = Greater?(x=w597, y=w604) -> (0:w598:bool)
                        n324 = Subtract(x=w597, y=w604) -> (x-y=w603:i32)
                        n325 = Absolute Value(x=w603) -> (abs(x)=w596:i32)
                        n326 = Multiply(x=w596, y=w595) -> (x*y=w594:i32)
                        n327 = for {
                          N: w594 -> [_]
                          tunnel: [w605] -> w593 mode=indexing
                          i -> [w606]
                          n328 = Increment(x=w606) -> (x+1=w608:i32)
                          n329 = Quotient & Remainder(x=w608, y=2) -> (x-y*floor(x/y)=w605:i32)  [unwired: 1 out]
                        }
                        n330 = To Double Precision Float(number=w593) -> (double precision float=w592:dbl[])
                        n331 = Delete From Array "Delete \nFrom Array"(array=w602, length=w594) -> (array with subset deleted=w601:dbl[])  [unwired: 1 in, 1 out]
                        n332 = Insert Into Array "Insert \nInto Array"(array=w602, new element=w592) -> (w599:dbl[])  [unwired: 1 in]
                        n333 = Select(t=w601, s=w598, f=w599) -> (s? t:f=w600:dbl[])
                      }
                      frame True {
                      }
                    }
                    n334 = In Range and Coerce(upper limit=w572, x=w573, lower limit=1) -> (coerced(x)=w576:i32)  [unwired: 1 out]
                    n335 = Multiply(x=w574, y=w576) -> (x*y=w577:i32)
                    n336 = To Unsigned Long Integer(number=w577) -> (unsigned 32bit integer=w575:u32)
                    n337 = To Variant(anything=w587) -> (Variant=w588:variant)
                    n338 = property class="Arr"(reference=w585, error in=w570, "Value"=w588, "Number of Rows"=w575) -> (error out=w584:errorcluster)  [unwired: 1 out]
                  }
                }
              }
            }
          }
          n339 = To Variant(anything=FALSE) -> (Variant=w474:variant)
          n340 = property class="Ctl"(reference=w475, error in=w473, "Value"=w474) -> (reference out=w471:refnum<vi>, error out=w469:errorcluster)
          n341 = Close Reference(reference=w471, error in (no error)=w469) -> (error out=w470:errorcluster)
        }
      }
    }
    frame Error {
    }
  }
  "Scale Error" <- w3
